vi "Save Library Documentation.vi"(9 "New Description":string, 10 "DQMH Modules Info In":T1, 11 "Library in":refnum<vi>) -> (0 "error out":errorcluster, 2 "DQMH Modules Info Out":T1, 3 "Lib out":refnum<vi>)   [LabVIEW 2019, in "Panther Dashboard.lvlib"]
uses:
  Panther Dashboard.lvlib
  DQMH Modules Info--cluster.ctl
  Module type--enum.ctl
  Project References--cluster.ctl
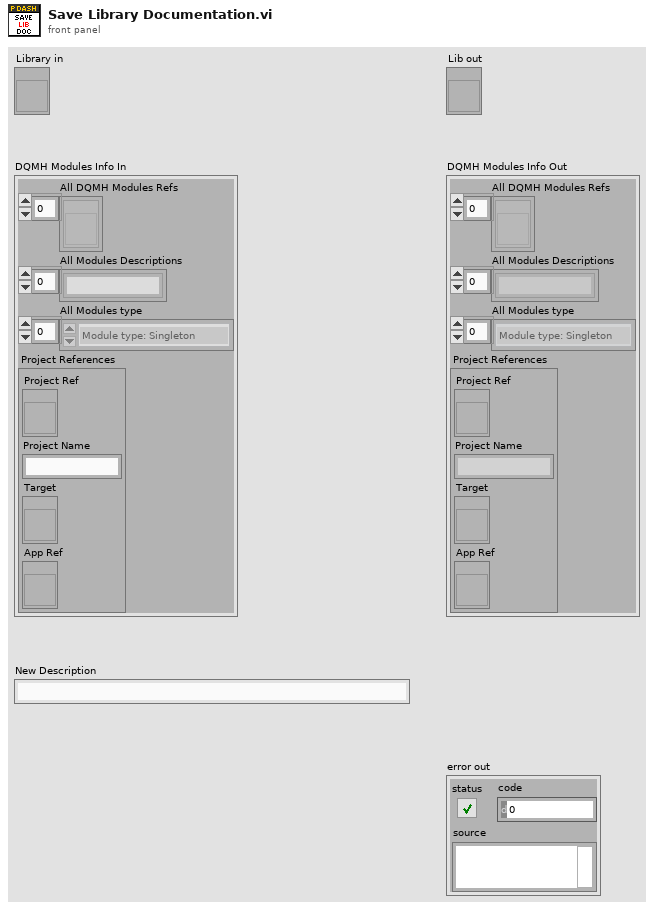
[diagram p1: front panel]
types:
  T1 = typedef "Panther Dashboard.lvlib/DQMH Modules Info--cluster.ctl" = cluster{"All DQMH Modules Refs":refnum<vi>[], "All Modules Descriptions":string[], "All Modules type":T2[], "Project References":T3}
  T2 = typedef "Panther Dashboard.lvlib/Module type--enum.ctl" = enum16{"Module type: Singleton", "Module type: Cloneable"}
  T3 = typedef "Panther Dashboard.lvlib/Project References--cluster.ctl" = cluster{"Project Ref":refnum<vi>, "Project Name":string, "Target":refnum<vi>, "App Ref":refnum<vi>}
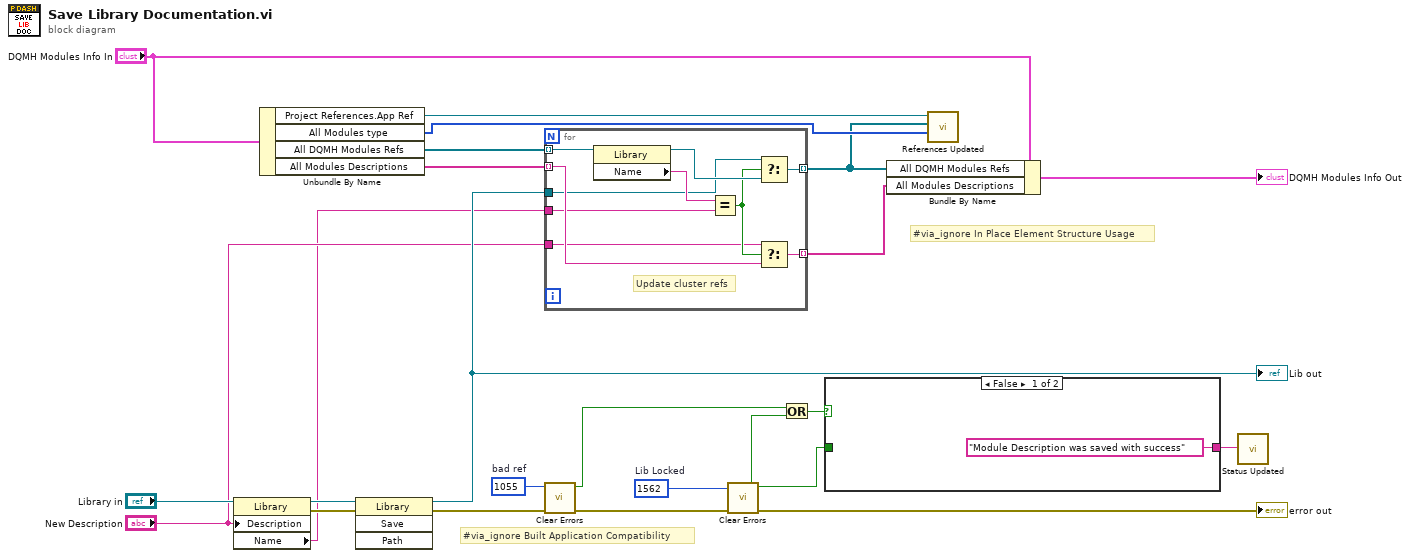
[diagram p0: block diagram]
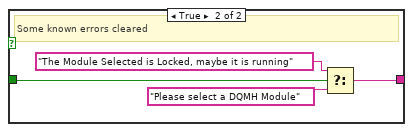
[diagram p2: hidden frame]
diagram:
  w7 = 1562  # Lib Locked
  w8 = 1055  # bad ref
  # "#via_ignore Built Application Compatibility"
  # "#via_ignore In Place Element Structure Usage"
  n1 = property class="Library"(reference="Library in", "Description"="New Description") -> (reference out=w17:refnum<vi>, error out=w23:errorcluster, "Name"=w10:string)  [unwired: 1 in]
  n2 = Unbundle By Name("DQMH Modules Info In") -> ("Project References.App Ref"=w2:refnum<vi>, "All Modules type"=w3:T2[], "All DQMH Modules Refs"=w18:refnum<vi>[], "All Modules Descriptions"=w13:string[])
  n3 = invoke class="Library" method="Save"(reference=w17, error in=w23) -> (reference out=w14:refnum<vi>, error out=w22:errorcluster)  [unwired: 2 in, 2 out]
  "Lib out" <- w14
  n4 = for {
    tunnel: w18 -> [w33] mode=indexing
    tunnel: [w30] -> w1 mode=indexing
    tunnel: w14 -> [w24]
    tunnel: w13 -> [w28] mode=indexing
    tunnel: [w27] -> w12 mode=indexing
    tunnel: "New Description" -> [w26]
    tunnel: w10 -> [w25]
    # "Update cluster refs"
    n5 = property class="Library"(reference=w33) -> (reference out=w31:refnum<vi>, "Name"=w32:string)  [unwired: 1 in, 1 out]
    n6 = Equal?(x=w32, y=w25) -> (x = y?=w29:bool)
    n7 = Select(t=w24, s=w29, f=w31) -> (s? t:f=w30:refnum<vi>)
    n8 = Select(t=w26, s=w29, f=w28) -> (s? t:f=w27:string)
  }
  n9 = call <vilib>:"Clear Errors.vi"("error in (no error)"=w22, "specific error code to clear (0: all)"=w8) -> ("error out"=w21:errorcluster, "specific error cleared?"=w9:bool)  [unwired: 4 in]
  n10 = call <vilib>:"Clear Errors.vi"("error in (no error)"=w21, "specific error code to clear (0: all)"=w7) -> ("error out"=→"error out":errorcluster, "specific error cleared?"=w5:bool)  [unwired: 4 in]
  n11 = Or(x=w9, y=w5) -> (x .or. y?=w6:bool)
  n12 = case shown="False" w6 {
    tunnel: w5 -> [_ w38]
    tunnel: ["Module Description was saved with success" ("Status") w35] -> w4
    frame False {
    }
    frame True {
      # "Some known errors cleared"
      n13 = Select(t="The Module Selected is Locked, maybe it is running" ("Status"), s=w38, f="Please select a DQMH Module" ("Status")) -> (s? t:f=w35:string)
    }
  }
  n14 = Bundle By Name(cluster="DQMH Modules Info In", "All DQMH Modules Refs"=w1, "All Modules Descriptions"=w12) -> (→"DQMH Modules Info Out":T1)
  n15 = call "References Updated.vi"("Modules Types"=w3, "Modules"=w1, "Application Instance"=w2) -> ()  [unwired: 8 in, 1 out]
  n16 = call "Status Updated.vi"("Status"=w4) -> ()  [unwired: 10 in, 1 out]
